vi "VFD-PC.vi"() -> ()   [LabVIEW 2017]
uses:
  <vilib>/Platform/TimedLoop/XDataNode/timing_clust.ctl
  <vilib>/Platform/TimedLoop/XDataNode/nitl_modes.ctl
  <vilib>/Platform/TimedLoop/XDataNode/wakeup.ctl
  <vilib>/NI Modbus.llb/MB Serial Master Query Write Single Register (poly).vi
  <vilib>/Platform/TimedLoop/XDataNode/XDataNode.xnode
  <vilib>/Platform/TimedLoop/XDataNode/XDNodeRunTimeDep.lvlib
  <vilib>/NI Modbus.llb/MB Serial Master Query Read Holding Registers (poly).vi
panel:
  in  "GS1 Communication Error In":errorcluster
  out "GS1 Communication Error Out":errorcluster
  out "Iteration Duration":i64
  out "Finished Late? [i-1]":bool
  out "TCHX Initializaton Error":errorcluster
  out "TCHX Initialization Loop Time (ms)":u32
  out "CTAH Initializaton Error":errorcluster
  out "CTAH Initialization Loop Time (ms)":u32
  out "Pump Initializaton Error":errorcluster
  out "Pump Initialization Loop Time (ms)":u32
  in  "Starting Address":u16
  out "Holding Registers":u16[](array[numeric])
  out "error out":errorcluster
  out "VISA resource name out":refnum<visa-resource-name>
  out "400001":u16
  out "error out":errorcluster
  # "Troubleshooting Modbus communication using third-party VIs and native I/O Server"
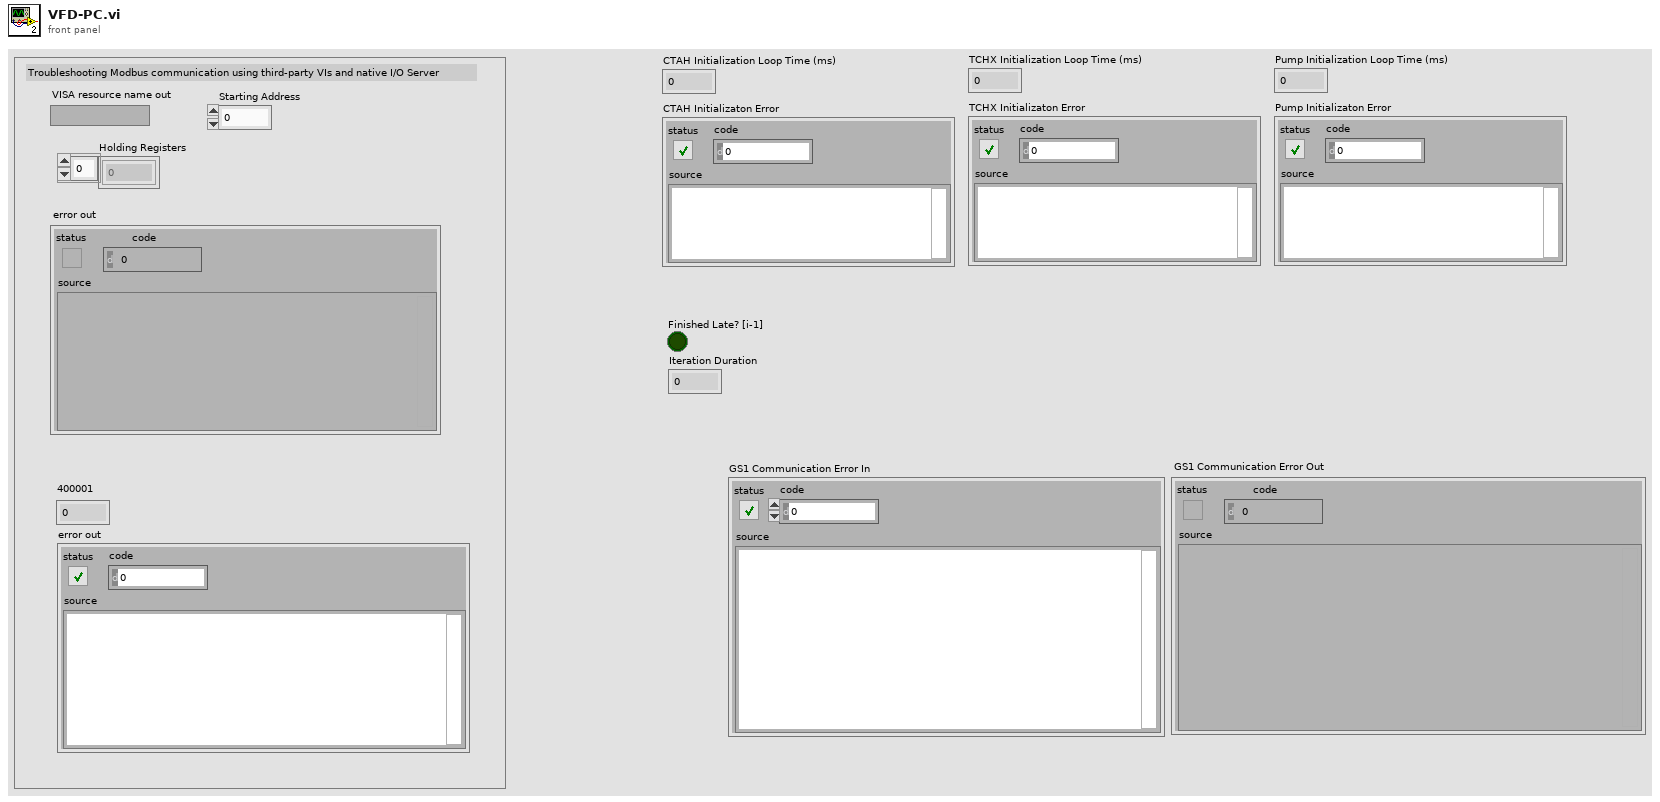
[diagram p1: front panel]
types:
  T1 = cluster{"Mode":enum16{"RTU", "ASCII"}, "Slave Address":u8}
  T2 = typedef "XDNodeRunTimeDep.lvlib/timing_clust.ctl" = cluster{"Expected End [f-1]":u64, "Actual End [f-1]":u64, "Finished Late? [f-1]":bool, "Expected End [i-1]":u64, "Actual End [i-1]":u64, "Finished Late? [i-1]":bool, "Expected Start [i]":u64, "Actual Start [i]":u64, "Expected Start [f]":u64, "Actual Start [f]":u64, "Source Name":string, "Structure Name":string, "Period":i64, "Deadline":i64, "Offset":i64, "Start":i64, "Priority":i32, "Timeout":i32, "Mode":T3, "Wakeup Reason":T4, "Error":errorcluster, "Source Type":string, "Secondary Source Type":string, "Global End Time":u64, "Global Start Time":u64, "Frame Duration":u64, "Iteration Duration":u64, "Assigned CPU":i32, "I/O Scan Engine Mode":u32}
  T3 = typedef "XDNodeRunTimeDep.lvlib/nitl_modes.ctl" = enum32{"No Change", "Process missed periods, maintain original phase", "Discard missed periods, maintain original phase", "Process missed periods, ignore original phase", "Discard missed periods, ignore original phase"}
  T4 = typedef "XDNodeRunTimeDep.lvlib/wakeup.ctl" = enum32{"Normal", "Aborted", "Asynchronous wakeup", "Timing source error", "Timed loop error", "Timeout"}
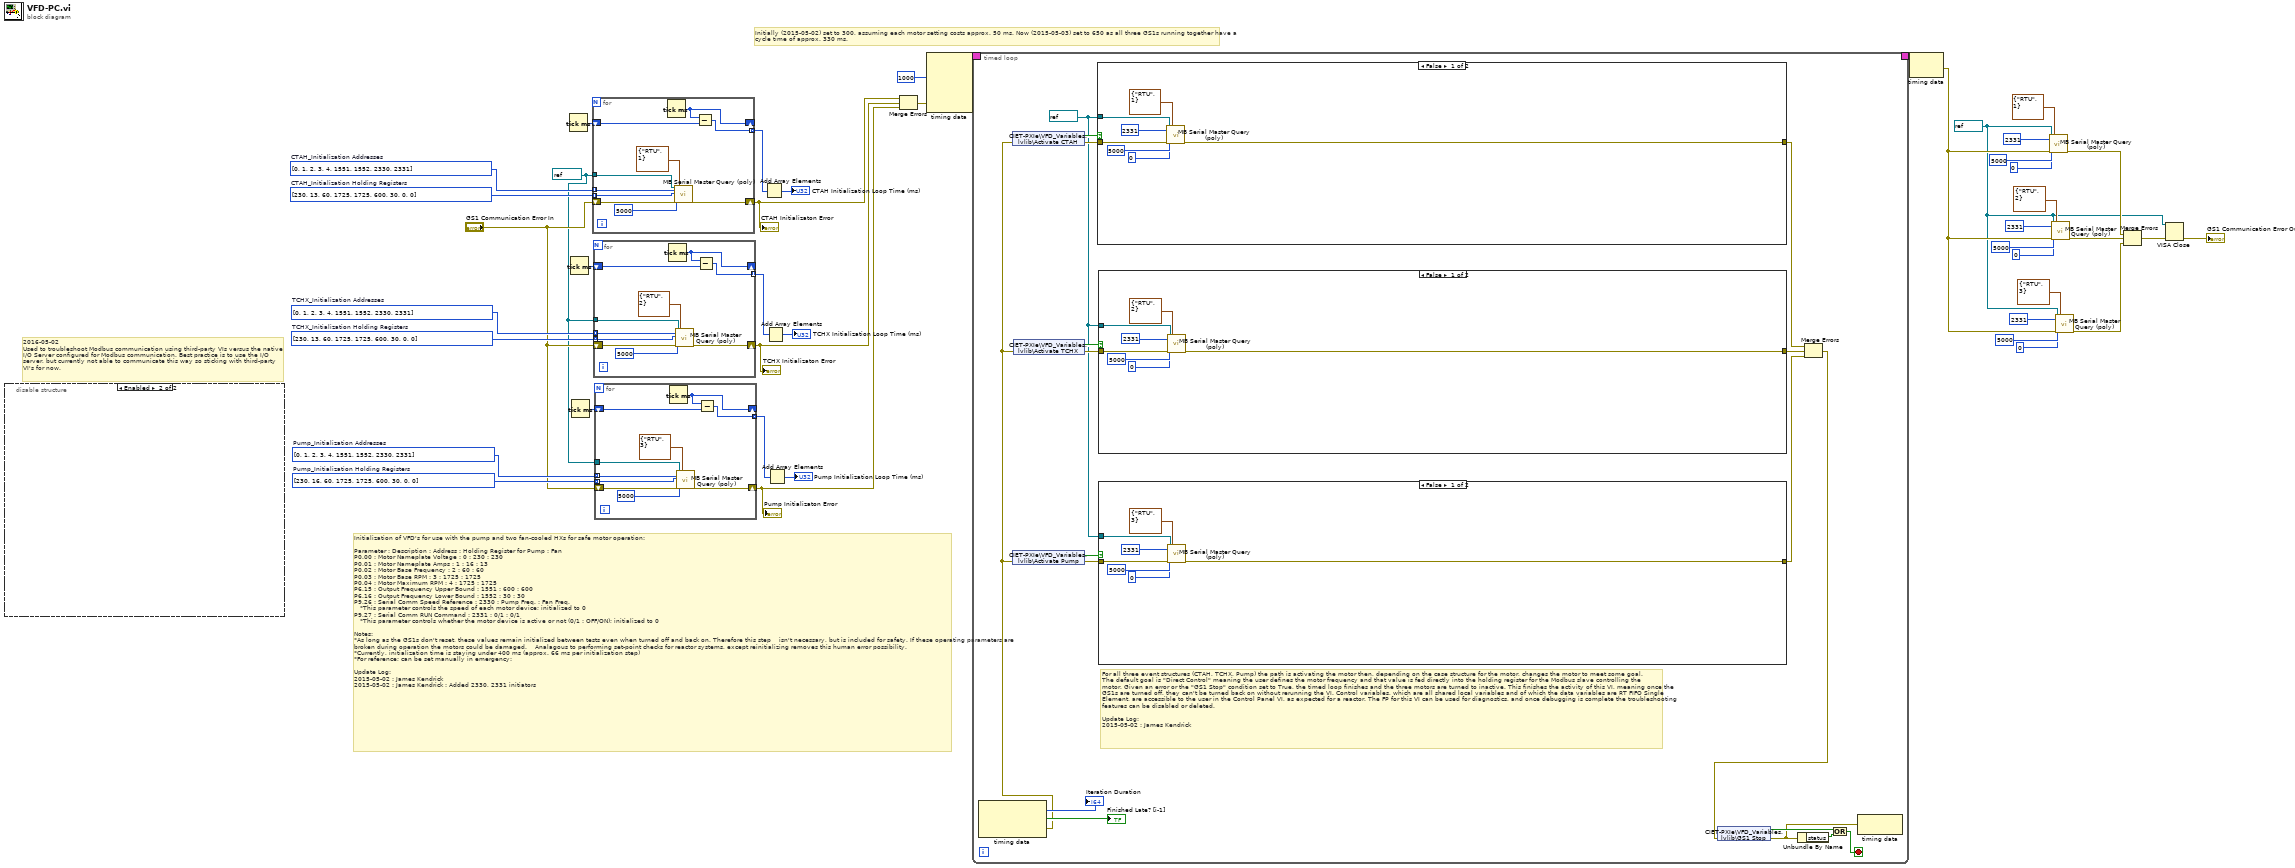
[diagram p0: block diagram]
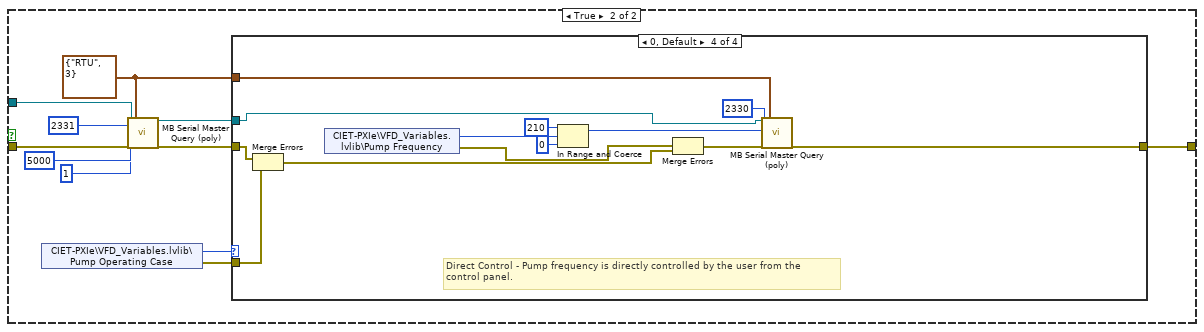
[diagram p2: hidden frame]
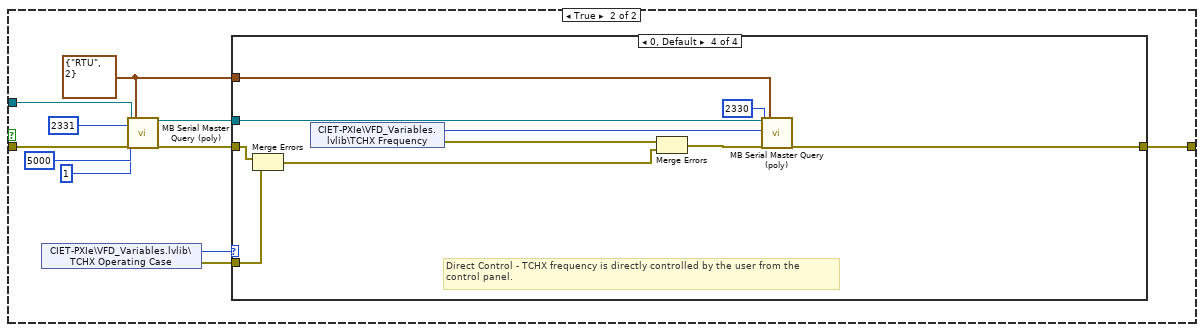
[diagram p6: hidden frame]
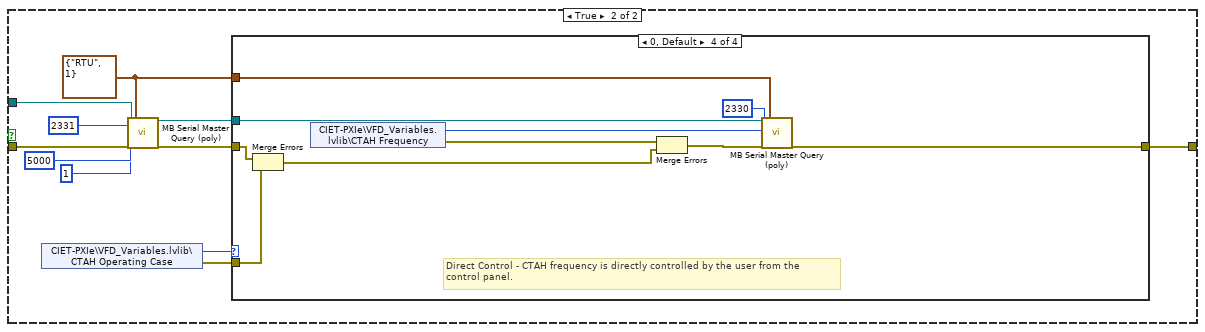
[diagram p10: hidden frame]
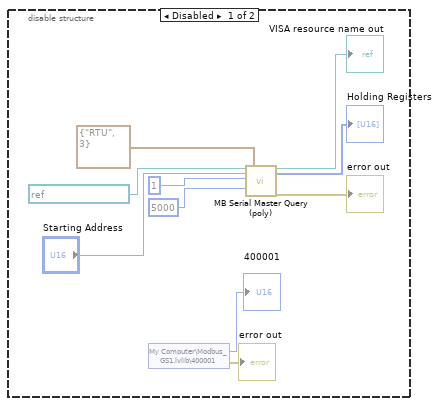
[diagram p14: hidden frame]
diagram:
  w1 = refnum<visa-resource-name> "VFD" ("VISA resource name")
  w7 = refnum<visa-resource-name> "VFD" ("VISA resource name")
  w29 = u16[] [230, 13, 60, 1725, 1725, 600, 30, 0, 0]  # TCHX_Initialization Holding Registers
  w30 = u16[] [0, 1, 2, 3, 4, 1551, 1552, 2330, 2331]  # TCHX_Initialization Addresses
  w34 = u16[] [230, 13, 60, 1725, 1725, 600, 30, 0, 0]  # CTAH_Initialization Holding Registers
  w35 = u16[] [0, 1, 2, 3, 4, 1551, 1552, 2330, 2331]  # CTAH_Initialization Addresses
  w42 = u16[] [230, 16, 60, 1725, 1725, 600, 30, 0, 0]  # Pump_Initialization Holding Registers
  w43 = u16[] [0, 1, 2, 3, 4, 1551, 1552, 2330, 2331]  # Pump_Initialization Addresses
  # "Initially (2015-05-02) set to 300, assuming each motor setting costs approx. 50 ms. Now (2015-05-03) set to 650 as all three GS1s running together have a \ncycle time of approx. 330 ms."
  # "2016-05-02\nUsed to troubleshoot Modbus communication using third-party VIs versus the native\nI/O Server configured for Modbus communication. Best practice is to use the I/O \nserver, but currently not able to communicate this way so sticking with third-party \nVI's for now."
  # "Initialization of VFD's for use with the pump and two fan-cooled HXs for safe motor operation:\n\nParameter : Description : Address : Holding Register for Pump : Fan\nP0.00 : Motor Nameplate Voltage : 0 : 230 : 230\nP0.01 : Motor Nameplate Amps : 1 : 16 : 13\nP0.02 : Motor Base Frequency : 2 : 60 : 60\nP0.03 : Motor Base RPM : 3 : 1725 : 1725\nP0.04 : Motor Maximum RPM : 4 : 1725 : 1725\nP6.15 : Output Frequency Upper Bound : 1551 : 600 : 600\nP6.16 : Output Frequency Lower Bound : 1552 : 30 : 30\nP9.26 : Serial Comm Speed Reference : 2330 : Pump Freq. : Fan Freq. \n   *This parameter controls the speed of each motor device; initialized to 0\nP9.27 : Serial Comm RUN Command : 2331 : 0/1 : 0/1\n   *This parameter controls whether the motor device is active or not (0/1 : OFF/ON); initialized to 0\n\nNotes:\n*As long as the GS1s don't reset, these values remain initialized between tests even when turned off and back on. Therefore this step    isn't necessary, but is included for safety. If these operating parameters are broken during operation the motors could be damaged.    Analagous to performing set-point checks for reactor systems, except reinitializing removes this human error possibility.\n*Currently, initialization time is staying under 400 ms (approx. 66 ms per initialization step)\n*For reference; can be set manually in emergency:\n\nUpdate Log:\n2015-05-02 : James Kendrick \n2015-05-02 : James Kendrick : Added 2330, 2331 initiators"
  n1 = disable-structure shown="Enabled" {
    frame Disabled {
      n2 = shared-variable "My Computer\\Modbus_GS1.lvlib\\400001"() -> (→"400001":u16, error out=→"error out":errorcluster)  [unwired: 1 in]
      n3 = call-poly <vilib>:"MB Serial Master Query (poly).vi"("VISA resource name"=refnum<visa-resource-name> "GS1_AC_Drive", "Starting Address"="Starting Address", "Quantity"=u16 1, "Timeout"=u32 5000, "Serial Parameters"=T1 {"Mode"=enum."RTU", "Slave Address"=3}) -> ("VISA resource name out"=→"VISA resource name out":refnum<visa-resource-name>, "Holding Registers"=→"Holding Registers":u16[], "error out"=→"error out":errorcluster)  [unwired: 11 in, 1 out]
    }
    frame Enabled {
    }
  }
  n4 = Tick Count (ms)() -> (millisecond timer value=w33:u32)
  n5 = Tick Count (ms)() -> (millisecond timer value=w28:u32)
  n6 = Tick Count (ms)() -> (millisecond timer value=w41:u32)
  n7 = for {
    shift-right: [w61] -> w14
    shift-left: "GS1 Communication Error In" -> [w62]
    tunnel: w35 -> [w60] mode=indexing
    tunnel: w34 -> [w59] mode=indexing
    shift-right: [w56] -> _
    shift-left: w33 -> [w58]
    tunnel: [w57] -> w32 mode=indexing
    tunnel: w7 -> [w55]
    n8 = Tick Count (ms)() -> (millisecond timer value=w56:u32)
    n9 = call-poly <vilib>:"MB Serial Master Query (poly).vi"("VISA resource name"=w55, "Address"=w60, "Holding Register"=w59, "Timeout"=u32 5000, "error in"=w62, "Serial Parameters"=T1 {"Mode"=enum."RTU", "Slave Address"=1}) -> ("error out"=w61:errorcluster)  [unwired: 11 in, 2 out]
    n10 = Subtract(x=w56, y=w58) -> (x-y=w57:u32)
  }
  "CTAH Initializaton Error" <- w14
  n11 = for {
    shift-right: [w71] -> w9
    shift-left: "GS1 Communication Error In" -> [w72]
    tunnel: w30 -> [w70] mode=indexing
    tunnel: w29 -> [w69] mode=indexing
    shift-right: [w66] -> _
    shift-left: w28 -> [w68]
    tunnel: [w67] -> w27 mode=indexing
    tunnel: w7 -> [w65]
    n12 = Tick Count (ms)() -> (millisecond timer value=w66:u32)
    n13 = call-poly <vilib>:"MB Serial Master Query (poly).vi"("VISA resource name"=w65, "Address"=w70, "Holding Register"=w69, "Timeout"=u32 5000, "error in"=w72, "Serial Parameters"=T1 {"Mode"=enum."RTU", "Slave Address"=2}) -> ("error out"=w71:errorcluster)  [unwired: 11 in, 2 out]
    n14 = Subtract(x=w66, y=w68) -> (x-y=w67:u32)
  }
  "TCHX Initializaton Error" <- w9
  n15 = for {
    shift-right: [w81] -> w8
    shift-left: "GS1 Communication Error In" -> [w82]
    tunnel: w43 -> [w80] mode=indexing
    tunnel: w42 -> [w79] mode=indexing
    shift-right: [w76] -> _
    shift-left: w41 -> [w78]
    tunnel: [w77] -> w40 mode=indexing
    tunnel: w7 -> [w75]
    n16 = Tick Count (ms)() -> (millisecond timer value=w76:u32)
    n17 = call-poly <vilib>:"MB Serial Master Query (poly).vi"("VISA resource name"=w75, "Address"=w80, "Holding Register"=w79, "Timeout"=u32 5000, "error in"=w82, "Serial Parameters"=T1 {"Mode"=enum."RTU", "Slave Address"=3}) -> ("error out"=w81:errorcluster)  [unwired: 11 in, 2 out]
    n18 = Subtract(x=w76, y=w78) -> (x-y=w77:u32)
  }
  "Pump Initializaton Error" <- w8
  n19 = Add Array Elements(numeric array=w32) -> (sum=→"CTAH Initialization Loop Time (ms)":u32)
  n20 = Add Array Elements(numeric array=w27) -> (sum=→"TCHX Initialization Loop Time (ms)":u32)
  n21 = Add Array Elements(numeric array=w40) -> (sum=→"Pump Initialization Loop Time (ms)":u32)
  n22 = Merge Errors(w14, w9, w8) -> (w16:errorcluster)
  n23 = node-c288(i64 1000 ("Pump Control Period (ms)"), w16) -> (w38:T2)  [unwired: 3 in]
  n24 = timed-loop {
    timing: w38 -> [_]
    timing-out: [_] -> w37
    stop <- w97 stop-if-true
    w84 = refnum<visa-resource-name> "VFD" ("VISA resource name")
    # "For all three event structures (CTAH, TCHX, Pump) the path is activating the motor then, depending on the case structure for the motor, changes the motor to meet some goal. \nThe default goal is \"Direct Control\" meaning the user defines the motor frequency and that value is fed directly into the holding register for the Modbus slave controlling the \nmotor. Given an error or the \"GS1 Stop\" condition set to True, the timed loop finishes and the three motors are turned to inactive. This finishes the activity of this VI, meaning once the\nGS1s are turned off, they can't be turned back on without rerunning the VI. Control variables, which are all shared local variables and of which the data variables are RT FIFO Single\nElement, are accessible to the user in the Control Panel VI, as expected for a reactor. The FP for this VI can be used for diagnostics, and once debugging is complete the troubleshooting\nfeatures can be disabled or deleted.  \n\nUpdate Log:\n2015-05-02 : James Kendrick"
    n25 = node-c288() -> (→"Iteration Duration":i64, →"Finished Late? [i-1]":bool, w90:errorcluster)  [unwired: 1 in]
    n26 = shared-variable "CIET-PXIe\\VFD_Variables.lvlib\\Activate CTAH"(error in=w90) -> (w101:bool, error out=w100:errorcluster)
    n27 = shared-variable "CIET-PXIe\\VFD_Variables.lvlib\\Activate Pump"(error in=w90) -> (w94:bool, error out=w93:errorcluster)
    n28 = shared-variable "CIET-PXIe\\VFD_Variables.lvlib\\Activate TCHX"(error in=w90) -> (w96:bool, error out=w95:errorcluster)
    n29 = case shown="False" w101 {
      tunnel: w100 -> [w164 w174]
      tunnel: [w163 w170] -> w88
      tunnel: w84 -> [w162 w169]
      frame False {
        n30 = call-poly <vilib>:"MB Serial Master Query (poly).vi"("VISA resource name"=w162, "Address"=u16 2331, "Holding Register"=u16 0, "Timeout"=u32 5000, "error in"=w164, "Serial Parameters"=T1 {"Mode"=enum."RTU", "Slave Address"=1}) -> ("error out"=w163:errorcluster)  [unwired: 11 in, 2 out]
      }
      frame True {
        w168 = T1 {"Mode"=enum."RTU", "Slave Address"=1} ("Serial Parameters")
        n31 = shared-variable "CIET-PXIe\\VFD_Variables.lvlib\\CTAH Operating Case"() -> (w172:i32, error out=w171:errorcluster)  [unwired: 1 in]
        n32 = call-poly <vilib>:"MB Serial Master Query (poly).vi"("VISA resource name"=w169, "Address"=u16 2331, "Holding Register"=u16 1, "Timeout"=u32 5000, "error in"=w174, "Serial Parameters"=w168) -> ("VISA resource name out"=w173:refnum<visa-resource-name>, "error out"=w175:errorcluster)  [unwired: 11 in, 1 out]
        n33 = case shown="0, Default" w172 {
          tunnel: w175 -> [_ _ _ w187]
          tunnel: w173 -> [_ _ _ w188]
          tunnel: w171 -> [_ _ _ w186]
          tunnel: [_ _ _ w180] -> w170
          tunnel: w168 -> [_ _ _ w179]
          frame 1 {
            # "CTAH Outlet Temp: Feedback - CTAH frequency is determined by a\ncontrol function to hold the outlet temperature of the CTAH \nconstant."
          }
          frame 2 {
            # "Load Following - CTAH frequency is controlled to make the CTAH heat removal power\nto equal a user specified value through satisfying the equation: m_dot*c_P*(T_in - T_out)"
          }
          frame 3 {
            # "Dynamic Forcing - CTAH frequency is defined by a waveform function to drive the \nCTAH frequency and thus mass flow rate in a dynamic pattern, such as a square wave,\nsine wave, or other function as defined by the user.\n\nUser inputs to include:\nCTAH frequency set point (used as signal offset)\nSignal amplitude\nSignal frequency\nSignal type: sine, square, others?"
          }
          frame 0, Default {
            # "Direct Control - CTAH frequency is directly controlled by the user from the\ncontrol panel."
            n34 = Merge Errors(w187, w186) -> (w181:errorcluster)
            n35 = shared-variable "CIET-PXIe\\VFD_Variables.lvlib\\CTAH Frequency"() -> (w184:u16, error out=w182:errorcluster)  [unwired: 1 in]
            n36 = Merge Errors(w182, w181) -> (w183:errorcluster)
            n37 = call-poly <vilib>:"MB Serial Master Query (poly).vi"("VISA resource name"=w188, "Address"=u16 2330, "Holding Register"=w184, "error in"=w183, "Serial Parameters"=w179) -> ("error out"=w180:errorcluster)  [unwired: 12 in, 2 out]
          }
        }
      }
    }
    n38 = case shown="False" w96 {
      tunnel: w95 -> [w136 w146]
      tunnel: [w135 w142] -> w86
      tunnel: w84 -> [w134 w141]
      frame False {
        n39 = call-poly <vilib>:"MB Serial Master Query (poly).vi"("VISA resource name"=w134, "Address"=u16 2331, "Holding Register"=u16 0, "Timeout"=u32 5000, "error in"=w136, "Serial Parameters"=T1 {"Mode"=enum."RTU", "Slave Address"=2}) -> ("error out"=w135:errorcluster)  [unwired: 11 in, 2 out]
      }
      frame True {
        w140 = T1 {"Mode"=enum."RTU", "Slave Address"=2} ("Serial Parameters")
        n40 = shared-variable "CIET-PXIe\\VFD_Variables.lvlib\\TCHX Operating Case"() -> (w144:i32, error out=w143:errorcluster)  [unwired: 1 in]
        n41 = call-poly <vilib>:"MB Serial Master Query (poly).vi"("VISA resource name"=w141, "Address"=u16 2331, "Holding Register"=u16 1, "Timeout"=u32 5000, "error in"=w146, "Serial Parameters"=w140) -> ("VISA resource name out"=w145:refnum<visa-resource-name>, "error out"=w147:errorcluster)  [unwired: 11 in, 1 out]
        n42 = case shown="0, Default" w144 {
          tunnel: w147 -> [_ _ _ w159]
          tunnel: w145 -> [_ _ _ w160]
          tunnel: w143 -> [_ _ _ w158]
          tunnel: [_ _ _ w152] -> w142
          tunnel: w140 -> [_ _ _ w151]
          frame 1 {
            # "TCHX Outlet Temp: Feedback - TCHX frequency is determined by a\ncontrol function to hold the outlet temperature of the TCHX \nconstant."
          }
          frame 2 {
            # "Freezing Event - TCHX frequency is adjust to simulate a freezing transient or freeze\nevent within the TCHX, compromising the heat transfer path from the core to\nenvironment during a transient without use of the pump/CTAH."
          }
          frame 3 {
            # "Dynamic Forcing - TCHX frequency is defined by a waveform function to drive the \nTCHX frequency and thus mass flow rate in a dynamic pattern, such as a square wave,\nsine wave, or other function as defined by the user.\n\nUser inputs to include:\nTCHX frequency set point (used as signal offset)\nSignal amplitude\nSignal frequency\nSignal type: sine, square, others?"
          }
          frame 0, Default {
            # "Direct Control - TCHX frequency is directly controlled by the user from the\ncontrol panel."
            n43 = Merge Errors(w159, w158) -> (w153:errorcluster)
            n44 = shared-variable "CIET-PXIe\\VFD_Variables.lvlib\\TCHX Frequency"() -> (w156:u16, error out=w154:errorcluster)  [unwired: 1 in]
            n45 = Merge Errors(w154, w153) -> (w155:errorcluster)
            n46 = call-poly <vilib>:"MB Serial Master Query (poly).vi"("VISA resource name"=w160, "Address"=u16 2330, "Holding Register"=w156, "error in"=w155, "Serial Parameters"=w151) -> ("error out"=w152:errorcluster)  [unwired: 12 in, 2 out]
          }
        }
      }
    }
    n47 = case shown="False" w94 {
      tunnel: w93 -> [w105 w115]
      tunnel: [w104 w111] -> w85
      tunnel: w84 -> [w103 w110]
      frame False {
        n48 = call-poly <vilib>:"MB Serial Master Query (poly).vi"("VISA resource name"=w103, "Address"=u16 2331, "Holding Register"=u16 0, "Timeout"=u32 5000, "error in"=w105, "Serial Parameters"=T1 {"Mode"=enum."RTU", "Slave Address"=3}) -> ("error out"=w104:errorcluster)  [unwired: 11 in, 2 out]
      }
      frame True {
        w109 = T1 {"Mode"=enum."RTU", "Slave Address"=3} ("Serial Parameters")
        n49 = shared-variable "CIET-PXIe\\VFD_Variables.lvlib\\Pump Operating Case"() -> (w113:i32, error out=w112:errorcluster)  [unwired: 1 in]
        n50 = call-poly <vilib>:"MB Serial Master Query (poly).vi"("VISA resource name"=w110, "Address"=u16 2331, "Holding Register"=u16 1, "Timeout"=u32 5000, "error in"=w115, "Serial Parameters"=w109) -> ("VISA resource name out"=w114:refnum<visa-resource-name>, "error out"=w116:errorcluster)  [unwired: 11 in, 1 out]
        n51 = case shown="0, Default" w113 {
          tunnel: w116 -> [_ _ _ w132]
          tunnel: w114 -> [_ _ _ w121]
          tunnel: w112 -> [_ _ _ w131]
          tunnel: [_ _ _ w127] -> w111
          tunnel: w109 -> [_ _ _ w120]
          frame 1 {
            # "Mass Flow Rate: Feedback - Pump frequency is controlled through \na closed feedback to match a specified mass flow rate defined by \nthe user on the control panel."
          }
          frame 2 {
            # "Mass Flow Rate: Ramp - Pump frequency is controlled through a control function that\ncontrols the rate of change of the mass flow rate that the user specifies on the control\npanel to match a user desired final mass flow rate."
          }
          frame 3 {
            # "Dynamic Forcing - Pump frequency is defined by a waveform function to drive the \npump frequency and thus mass flow rate in a dynamic pattern, such as a square wave,\nsine wave, or other function as defined by the user.\n\nUser inputs to include:\nPump frequency set point (used as signal offset)\nSignal amplitude\nSignal frequency\nSignal type: sine, square, others?"
          }
          frame 0, Default {
            # "Direct Control - Pump frequency is directly controlled by the user from the\ncontrol panel."
            n52 = Merge Errors(w132, w131) -> (w128:errorcluster)
            n53 = shared-variable "CIET-PXIe\\VFD_Variables.lvlib\\Pump Frequency"() -> (w124:u16, error out=w122:errorcluster)  [unwired: 1 in]
            n54 = In Range and Coerce(upper limit=u16 210, x=w124, lower limit=u16 0) -> (coerced(x)=w123:u16)  [unwired: 1 out]
            n55 = Merge Errors(w122, w128) -> (w129:errorcluster)
            n56 = call-poly <vilib>:"MB Serial Master Query (poly).vi"("VISA resource name"=w121, "Address"=u16 2330, "Holding Register"=w123, "error in"=w129, "Serial Parameters"=w120) -> ("error out"=w127:errorcluster)  [unwired: 12 in, 2 out]
          }
        }
      }
    }
    n57 = Merge Errors(w88, w86, w85) -> (w87:errorcluster)
    n58 = shared-variable "CIET-PXIe\\VFD_Variables.lvlib\\GS1 Stop"(error in=w87) -> (w92:bool, error out=w89:errorcluster)
    n59 = Unbundle By Name(w89) -> ("status"=w91:bool)
    n60 = Or(x=w92, y=w91) -> (x .or. y?=w97:bool)
    n61 = node-c288(w89) -> ()  [unwired: 1 out]
  }
  n62 = node-c288(w37) -> (w10:errorcluster)
  n63 = call-poly <vilib>:"MB Serial Master Query (poly).vi"("VISA resource name"=w1, "Address"=u16 2331, "Holding Register"=u16 0, "Timeout"=u32 5000, "error in"=w10, "Serial Parameters"=T1 {"Mode"=enum."RTU", "Slave Address"=1}) -> ("error out"=w12:errorcluster)  [unwired: 11 in, 2 out]
  n64 = call-poly <vilib>:"MB Serial Master Query (poly).vi"("VISA resource name"=w1, "Address"=u16 2331, "Holding Register"=u16 0, "Timeout"=u32 5000, "error in"=w10, "Serial Parameters"=T1 {"Mode"=enum."RTU", "Slave Address"=2}) -> ("error out"=w13:errorcluster)  [unwired: 11 in, 2 out]
  n65 = call-poly <vilib>:"MB Serial Master Query (poly).vi"("VISA resource name"=w1, "Address"=u16 2331, "Holding Register"=u16 0, "Timeout"=u32 5000, "error in"=w10, "Serial Parameters"=T1 {"Mode"=enum."RTU", "Slave Address"=3}) -> ("error out"=w11:errorcluster)  [unwired: 11 in, 2 out]
  n66 = Merge Errors(w12, w13, w11) -> (w2:errorcluster)
  n67 = VISA Close(VISA resource name=w1, error in (no error)=w2) -> (error out=→"GS1 Communication Error Out":errorcluster)
